vi "Save_energy.vi"(9 "Voltage":dbl[](array[numeric]), 10 "Time":dbl[](array[numeric]), 11 "file path":path=path "C:/Projects/MPE_analyzer/Signal.csv") -> (3 "output array":dbl[][](array[numeric]))   [LabVIEW 2018]
uses:
  <vilib>/Utility/file.llb/Write Delimited Spreadsheet (DBL).vi
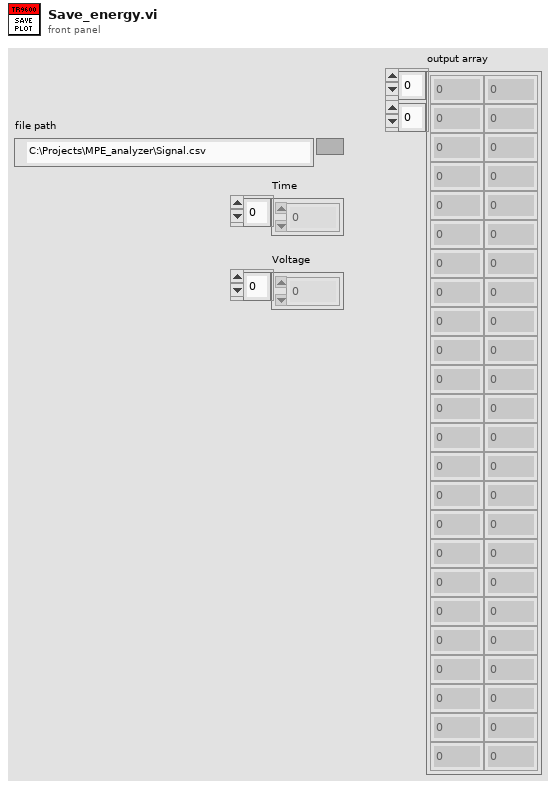
[diagram p1: front panel]
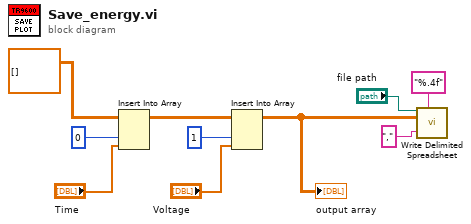
[diagram p0: block diagram]
diagram:
  n1 = Insert Into Array(array=dbl[][] [] ("Array"), index (col)=0 ("disabled index (col)"), new element="Time") -> (w2:dbl[][])  [unwired: 1 in]
  n2 = Insert Into Array(array=w2, index (col)=1 ("disabled index (col)"), new element="Voltage") -> (w5:dbl[][])  [unwired: 1 in]
  "output array" <- w5
  n3 = call-poly <vilib>:"Write Delimited Spreadsheet.vi"("file path (dialog if empty)"="file path", "format (%.3f)"="%.4f", "2D data"=w5, "delimiter (\\t)"="," ("delimiter (\\t)")) -> ()  [unwired: 10 in, 2 out]
